vi "Sample_Test.vi"(8 "error in (no error)":errorcluster) -> (0 "error out":errorcluster, 3 "Test Passed":bool)   [LabVIEW 2019]
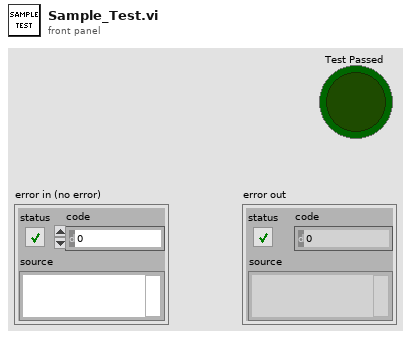
[diagram p1: front panel]
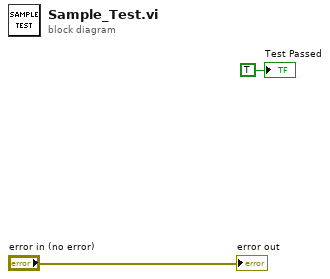
[diagram p0: block diagram]
diagram:
  "error out" <- "error in (no error)"
  "Test Passed" <- TRUE ("Test Passed")
